vi "Write Reply Notifier.vi"(8 "error in (no error)":errorcluster, 10 "Reply Notifier":refnum<notifier>, 11 "29-Equipment Requests Time Value from Host in":refnum<class "29-Equipment Requests Time Value from Host.lvclass">) -> (0 "error out":errorcluster, 3 "29-Equipment Requests Time Value from Host out":refnum<class "29-Equipment Requests Time Value from Host.lvclass">)   [LabVIEW 2020, in "SECS Scenarios.lvlib" / "29-Equipment Requests Time Value from Host.lvclass"]
uses:
  29-Equipment Requests Time Value from Host.lvclass
  29-Equipment Requests Time Value from Host.lvclass/29-Equipment Requests Time Value from Host.ctl
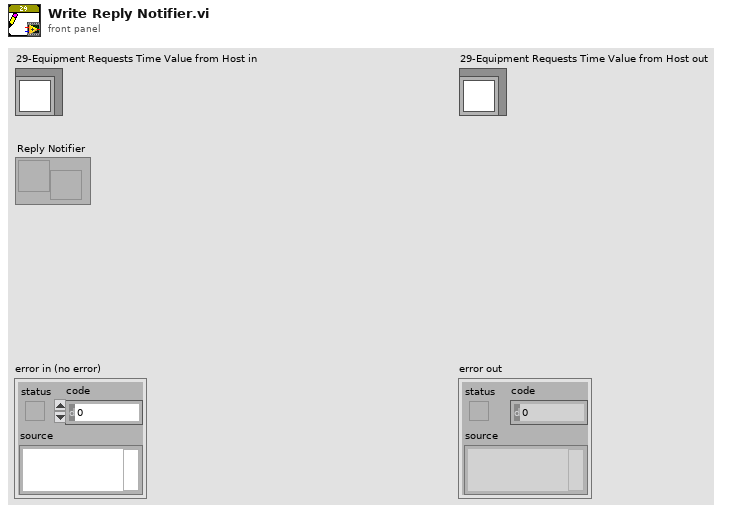
[diagram p1: front panel]
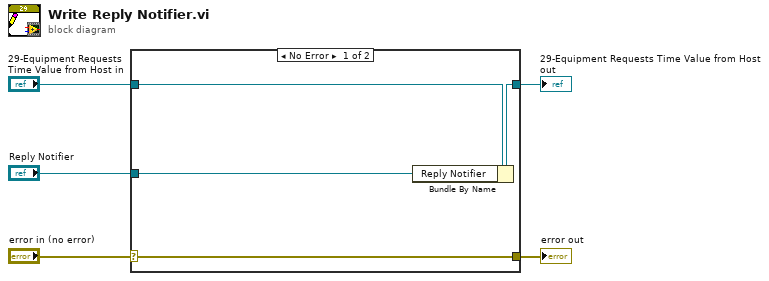
[diagram p0: block diagram]
diagram:
  n1 = case shown="No Error" "error in (no error)" {
    selector: "error in (no error)" -> [w9 w10]
    tunnel: [w9 w10] -> w4
    tunnel: [w7 w11] -> w2
    tunnel: "29-Equipment Requests Time Value from Host in" -> [w8 w11]
    tunnel: "Reply Notifier" -> [w6 _]
    frame No Error {
      n2 = Bundle By Name(cluster=w8, "Reply Notifier"=w6) -> (w7:refnum<class "29-Equipment Requests Time Value from Host.lvclass">)
    }
    frame Error {
    }
  }
  "error out" <- w4
  "29-Equipment Requests Time Value from Host out" <- w2
